vi "write_other_randoms.vi"() -> ()   [LabVIEW 2018]
panel:
  out "Dynamic Data Type":dynamicdata(graph)
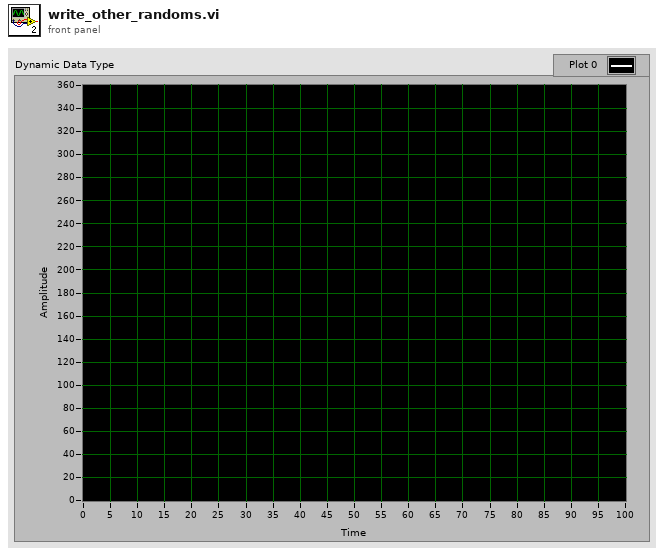
[diagram p1: front panel]
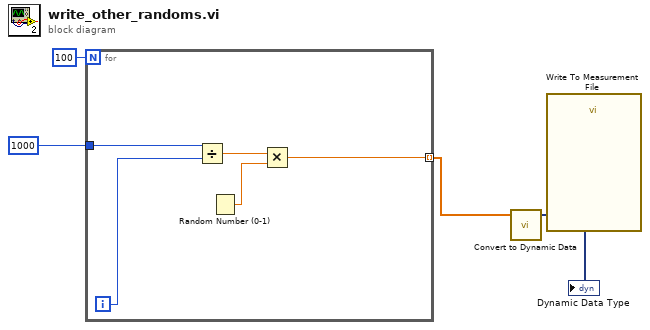
[diagram p0: block diagram]
diagram:
  n1 = for {
    N: 100 -> [_]
    tunnel: 1000 -> [w9]
    tunnel: [w5] -> w2 mode=indexing
    i -> [w8]
    n2 = Divide(x=w9, y=w8) -> (x/y=w7:dbl)
    n3 = Random Number (0-1)() -> (number: 0 to 1=w6:dbl)
    n4 = Multiply(x=w7, y=w6) -> (x*y=w5:dbl)
  }
  n5 = call "Convert to Dynamic Data"("Array"=w2) -> ("Dynamic Data Type"=w1:dynamicdata)  [unwired: 3 in]
  "Dynamic Data Type" <- w1
  n6 = call "Write To Measurement File"("Signals"=w1) -> ()  [unwired: 16 in, 3 out]
